vi "IrDA Date Client.vi"(2 "error in (no error)":errorcluster, 4 "IrDA Refnum":refnum<k19>) -> (1 "Data Received":string)   [LabVIEW 2011]
doc: "Reads the date and time sent from the Date Server VI in this LLB. The VI first reads 4 bytes defining the length of the date string, then reads the date. After you click the stop button, this VI sends a single character to tell the Date Server VI to terminate."
panel:
  in  "stop":bool
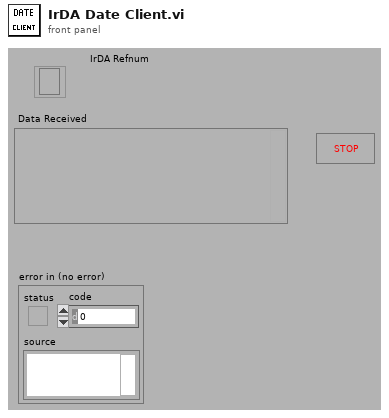
[diagram p1: front panel]
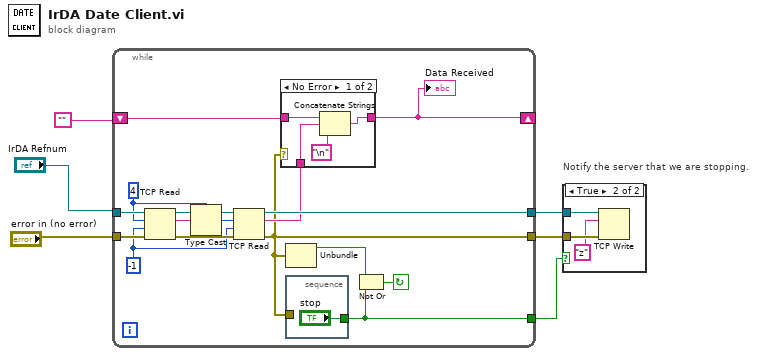
[diagram p0: block diagram]
diagram:
  n1 = while {
    tunnel: [w11] -> w4
    tunnel: [w15] -> w6
    tunnel: [w7] -> w5
    tunnel: "error in (no error)" -> [w21]
    tunnel: "IrDA Refnum" -> [w22]
    shift-right: [w8] -> _
    shift-left: "" -> [w10]
    stop <- w12 continue-if-true
    w14 = -1
    w20 = 4
    n2 = TCP Read(connection ID=w22, bytes to read=w20, error in (no error)=w21, 9:w14) -> (connection ID out=w16:refnum<k19>, data out=w19:string, error out=w18:errorcluster)  [unwired: 1 out]
    n3 = Type Cast(type=w20, x=w19) -> (*(type *) &x=w17:i32)
    n4 = TCP Read(connection ID=w16, bytes to read=w17, error in (no error)=w18, 9:w14) -> (connection ID out=w15:refnum<k19>, data out=w9:string, error out=w7:errorcluster)  [unwired: 1 out]
    n5 = case shown="No Error" w7 {
      tunnel: w10 -> [w26 w27]
      tunnel: w9 -> [w25 _]
      tunnel: [w23 w27] -> w8
      frame No Error {
        n6 = Concatenate Strings(w26, w25, "\n") -> (w23:string)
      }
      frame Error {
      }
    }
    "Data Received" <- w8
    n7 = Unbundle(w7) -> ("status"=w13:bool)  [unwired: 2 out]
    n8 = stacked-sequence {
      tunnel: w7 -> [_]
      tunnel: ["stop"] -> w11
      frame #0 {
      }
    }
    n9 = Not Or(1:w11, 2:w13) -> (0:w12:bool)
  }
  n10 = case "Notify the server that we are stopping." shown="True" w4 {
    tunnel: w6 -> [_ w31]
    tunnel: w5 -> [_ w30]
    frame False {
    }
    frame True {
      n11 = TCP Write(connection ID=w31, data in="z", error in (no error)=w30) -> ()  [unwired: 4 out]
    }
  }
